vi "amplitudeScanDone.vi"(8 "error in (no error)":errorcluster, 11 "Model in":refnum<class "Model.lvclass">) -> (0 "error out":errorcluster, 2 "Done?":bool, 3 "Model out":refnum<class "Model.lvclass">)   [LabVIEW 2015]
uses:
  Model.lvclass
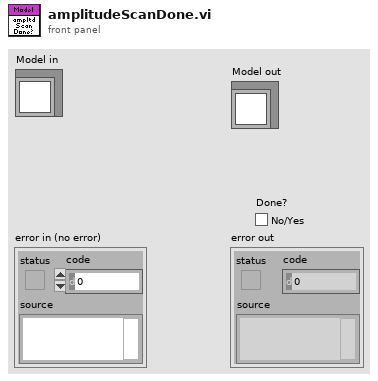
[diagram p1: front panel]
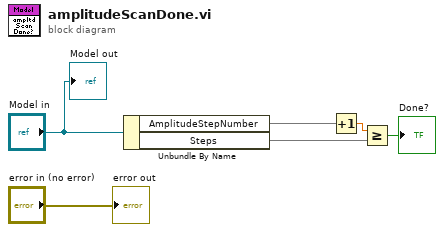
[diagram p0: block diagram]
diagram:
  n1 = Unbundle By Name("Model in") -> ("AmplitudeStepNumber"=w3, "Steps"=w1)
  n2 = Increment(x=w3) -> (x+1=w2:dbl)
  n3 = Greater Or Equal?(x=w2, y=w1) -> (x >= y?=→"Done?":bool)
  "error out" <- "error in (no error)"
  "Model out" <- "Model in"
